vi "Run.vi"(8 "error in (no error)":errorcluster, 11 "SaveWaveforms in":refnum<class "SaveWaveforms.lvclass">) -> (0 "error out":errorcluster, 2 "TimeOut":bool, 3 "SaveWaveforms out":refnum<class "SaveWaveforms.lvclass">)   [LabVIEW 2018, in "AnalysisPlugins.lvlib" / "SaveWaveforms.lvclass"]
uses:
  SaveWaveforms.lvclass
  X:/Projects/PMUCal/Modules/Analysis/AnalysisPlugins/AnalysisPluginBaseClass/AnalysisPluginsBase.lvclass
  AnalysisPluginBaseClass/Typedefs/SampleDataInput.ctl
  AnalysisPluginBaseClass/AnalysisPluginsBase.lvclass/AnalysisPluginsBase.ctl
  AnalysisPluginBaseClass/Accessors/Read SampleDataQueName.vi
  AnalysisPluginBaseClass/AnalysisPluginsBase.lvclass
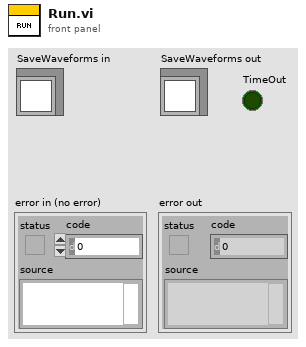
[diagram p1: front panel]
types:
  T1 = typedef "AnalysisPlugins.lvlib/AnalysisPluginsBase.lvclass/SampleDataInput.ctl" = waveform(dbl)[]
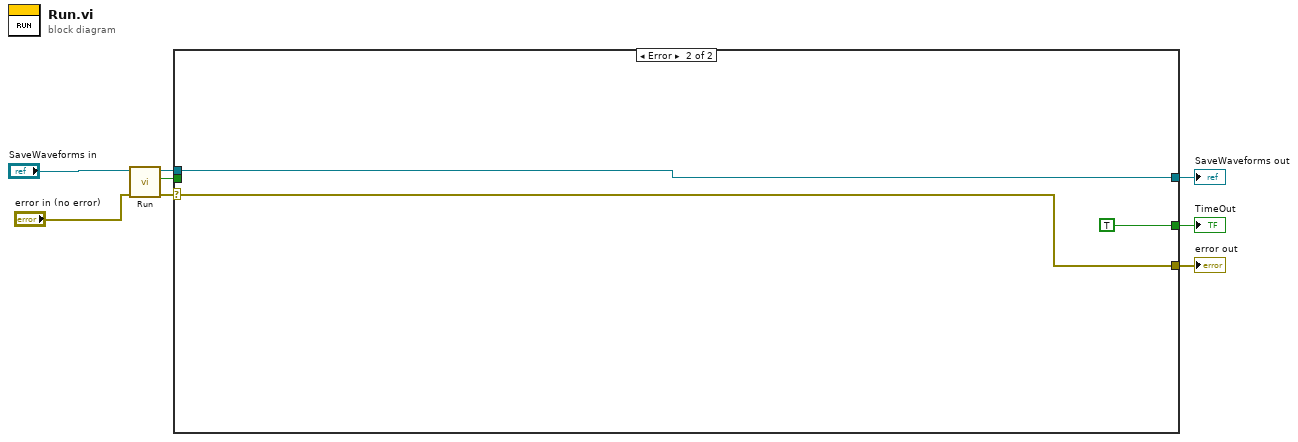
[diagram p0: block diagram]
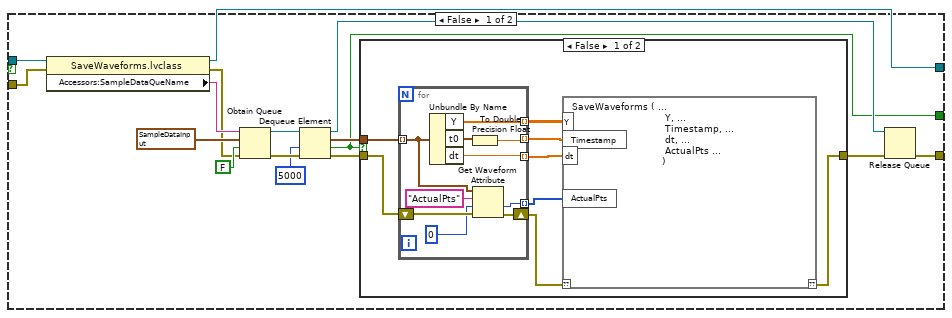
[diagram p3: hidden frame]
diagram:
  n1 = call-parent "Run.vi"("error in (no error)"="error in (no error)", "AnalysisPluginsBase in"="SaveWaveforms in") -> ("error out"=w6:errorcluster, "TimeOut"=w1:bool, "AnalysisPluginsBase out"=w5:refnum<class "SaveWaveforms.lvclass">)  [unwired: 7 in]
  n2 = case shown="Error" w6 {
    selector: w6 -> [w13 w55]
    tunnel: w5 -> [w14 w54]
    tunnel: [w12 w55] -> w4
    tunnel: [w11 w54] -> w3
    tunnel: [w10 TRUE] -> w2
    tunnel: w1 -> [w9 _]
    frame No Error {
      n3 = case shown="True" w9 {
        selector: w9 -> [_ w51]
        tunnel: w14 -> [w30 w52]
        tunnel: w13 -> [w29 w50]
        tunnel: [w17 w50] -> w12
        tunnel: [w16 w52] -> w11
        tunnel: [w15 w51] -> w10
        frame False {
          n4 = property class="SaveWaveforms.lvclass"(reference=w30, error in=w29) -> (reference out=w16:refnum<class "SaveWaveforms.lvclass">, error out=w25:errorcluster, "Accessors:SampleDataQueName"=w28:string)
          n5 = Obtain Queue(name (unnamed)=w28, element data type=T1 [{"t0"=timestamp(0 s since 1904-01-01), "dt"=1.0, "Y"=[]}] ("clSampleDataArray"), create if not found? (T)=FALSE, error in (no error)=w25) -> (queue out=w23:refnum<queue>, error out=w24:errorcluster)  [unwired: 1 in, 1 out]
          n6 = Dequeue Element(queue=w23, timeout in ms (-1)=5000, error in (no error)=w24) -> (queue out=w18:refnum<queue>, element=w20:T1, timed out?=w15:bool, error out=w21:errorcluster)
          n7 = case shown="False" w15 {
            tunnel: w21 -> [w37 w49]
            tunnel: w20 -> [w38 _]
            tunnel: [w31 w49] -> w19
            frame False {
              n8 = for {
                tunnel: w38 -> [w46] mode=indexing
                tunnel: [w39] -> w34 mode=indexing
                tunnel: [w40] -> w35 mode=indexing
                tunnel: [w48] -> w36 mode=indexing
                shift-right: [w44] -> w32
                shift-left: w37 -> [w45]
                tunnel: [w42] -> w33 mode=indexing
                n9 = Unbundle By Name(w46) -> ("Y"=w48:dbl[], "t0"=w41:timestamp, "dt"=w39:dbl)
                n10 = To Double Precision Float(number=w41) -> (double precision float=w40:dbl)
                n11 = Get Waveform Attribute(4:w45, 5:0, 6:"ActualPts" ("name"), 7:w46) -> (0:w44:errorcluster, 1:w42:i32)  [unwired: 2 out]
              }
              n12 = script code="SaveWaveforms ( ...\n                               Y, ...\n                               Timestamp, ...\n                               dt, ...\n                               ActualPts ...\n                              )"("??"=w32, "Y"=w36, "Timestamp"=w35, "dt"=w34, "ActualPts"=w33) -> ("??"=w31:errorcluster)
            }
            frame True {
            }
          }
          n13 = Release Queue(queue=w18, error in (no error)=w19) -> (error out=w17:errorcluster)  [unwired: 1 in, 2 out]
        }
        frame True {
        }
      }
    }
    frame Error {
    }
  }
  "error out" <- w4
  "SaveWaveforms out" <- w3
  "TimeOut" <- w2
